vi "多参数传感器参数读取.vi"(8 "Error in":errorcluster caption="Error in (no error)") -> (0 "error out":errorcluster, 3 "添加的数组":string[][](array[string]))   [LabVIEW 2016, in "斯坦道仪器.lvlib"]
panel:
  in  "下拉列表":u16(ring) items=["氨氮"=3, "水温"=9, "pH"=10, "溶解氧"=11, "电导率"=12, "浊度"=13, "叶绿素a"=14, "藻密度"=15, "蓝绿藻"=16, "氧化还原电位"=17, "溶解氧%"=18, "盐度"=19, "水中油"=20, "高锰酸盐指数"=21, "化学需氧量"=22, "比电导率"=23, "总溶解固体"=24, "pH电极电位"=25]
  in  "传感器区":i32(listbox)
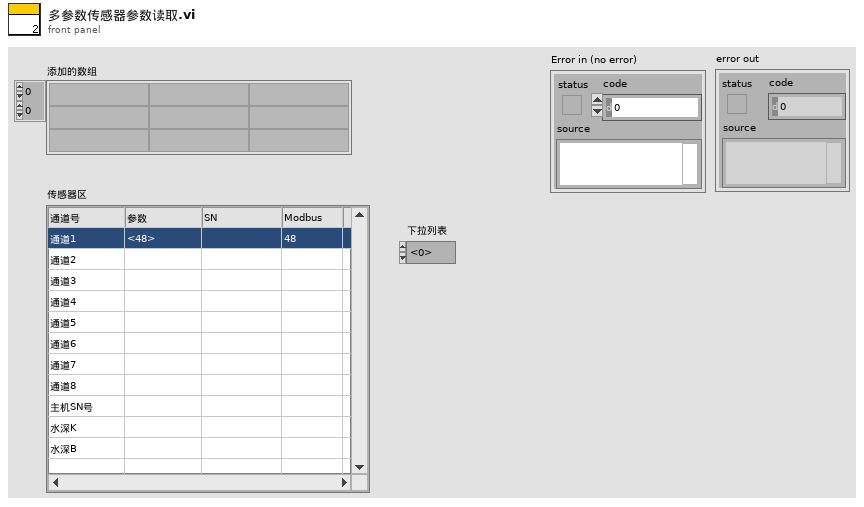
[diagram p1: front panel]
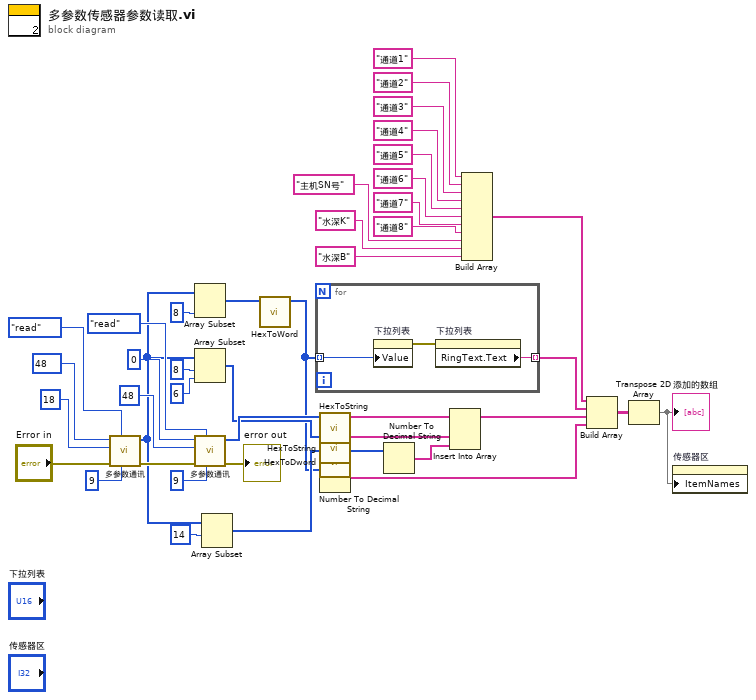
[diagram p0: block diagram]
diagram:
  n1 = call "多参数通讯.vi"("Slave ID"=u8 9, "STEP"=enum16{"open", "read", "write", "close"}."read", "Error in"="Error in", "quantity"=u16 18, "starting address"=u16 48) -> ("error out"=w21:errorcluster, "Registers"=w14:u16[])  [unwired: 4 in, 1 out]
  n2 = Array Subset(array=w14, length=8 ("长度")) -> (w17:u16[])  [unwired: 1 in]
  n3 = Array Subset(array=w14, index=8 ("索引"), length=6 ("长度")) -> (w12:u16[])
  n4 = call "多参数通讯.vi"("Slave ID"=u8 9, "STEP"=enum16{"open", "read", "write", "close"}."read", "Error in"=w21, "quantity"=u16 48, "starting address"=u16 0) -> ("error out"=→"error out":errorcluster, "Registers"=w38:u16[])  [unwired: 4 in, 1 out]
  n5 = Array Subset(array=w14, index=14 ("索引")) -> (w4:u16[])  [unwired: 1 in]
  n6 = call "HexToWord.vi"("数组"=w17) -> ("WORD"=w2:u16[])  [unwired: 10 in]
  n7 = for {
    tunnel: w2 -> [w44] mode=indexing
    tunnel: [w43] -> w19 mode=indexing
    n8 = property on="下拉列表" class="Ring (严格)"("Value"=w44) -> (error out=w45:errorcluster)  [unwired: 2 in, 1 out]
    n9 = property on="下拉列表" class="Ring (严格)"(error in=w45) -> ("RingText.Text"=w43:string)  [unwired: 1 in, 2 out]
  }
  n10 = call "HexToString.vi"("数组"=w38) -> ("STRING"=w11:string[])  [unwired: 10 in]
  n11 = call "HexToString.vi"("数组"=w12) -> ("STRING"=w10:string[])  [unwired: 10 in]
  n12 = call "HexToDword.vi"("数组"=w4) -> ("DWORD"=w3:i32[])  [unwired: 10 in]
  n13 = Number To Decimal String(number=w2) -> (decimal integer string=w1:string[])  [unwired: 1 in]
  n14 = Number To Decimal String(number=w3) -> (decimal integer string=w9:string[])  [unwired: 1 in]
  n15 = Insert Into Array(array=w11, new element #1=w10, new element #2=w9) -> (w8:string[])  [unwired: 1 in]
  n16 = Build Array("通道1", "通道2", "通道3", "通道4", "通道5", "通道6", "通道7", "通道8", "主机SN号", "水深K", "水深B") -> (w29:string[])
  n17 = Build Array(w29, w19, w8, w1) -> (w28:string[][])
  n18 = Transpose 2D Array(2D array=w28) -> (transposed array=w27:string[][])
  "添加的数组" <- w27
  n19 = property on="传感器区" class="MCListbox (严格)"("ItemNames"=w27) -> ()  [unwired: 2 in, 2 out]
